vi "MT Compensate Sample Clock Frequency Error (QAM).vi"(0 "input complex waveform":T1={"t0"=0.0, "dt"=1.0, "Y"=[]} {"Y" format="%.3f"; "dt" format="%^.2e"; "t0" format="%.4f"}, 5 "samples per symbol":i32=16, 7 "matched filter coefficients":dbl[](array[numeric]), 9 "clock phase computation window (symbols)":i32=256, 11 "error in (no error)":errorcluster) -> (4 "output complex waveform":T1 {"Y" format="%.3f"; "dt" format="%^.2e"; "t0" format="%.4f"}, 6 "sample clock frequency error (ppm)":dbl, 15 "error out":errorcluster)   [LabVIEW 2020, in "niDMT.lvlib"]
doc: "This polymorphic instance corrects the sample clock frequency offset before calling the MT Demodulate QAM VI."
uses:
  <vilib>/addons/Modulation/niDMT.lvlib
  <vilib>/addons/Modulation/Analog/controls/Complex Data Waveform.ctl
  <vilib>/Analysis/baseanly.llb/Mean (DBL).vi
  <vilib>/addons/Modulation/Analog/support/Validators/mod_Fractional Resample Validate.vi
  <vilib>/addons/Modulation/Analog/support/Validators/mod_Check Flush State.vi
  <vilib>/addons/Modulation/Analog/support/mod_FractionalResampler.vi
  <vilib>/addons/Modulation/Analog/support/mod_Integer Rate Interpolation.vi
  <vilib>/addons/Modulation/Analog/support/mod_Set Error Source.vi
  <vilib>/addons/Modulation/Analog/support/Validators/mod_WFErrorHandler.vi
  <vilib>/addons/Modulation/Analog/support/mod_PerformResampling.vi
  <vilib>/Utility/error.llb/Error Cluster From Error Code.vi
  <vilib>/addons/Modulation/Analog/support/mod_Resampling Factors.vi
  <vilib>/addons/Modulation/Analog/support/mod_ResamplingFilter.vi
  <vilib>/addons/Modulation/Analog/support/mod_Generate Integer Interpolation Filter.vi
  <vilib>/addons/Modulation/Digital/General/MT Apply Matched Filter (Generic).vi
  <vilib>/addons/Modulation/niAMT.lvlib
  <vilib>/Analysis/NI_AALPro.lvlib
  <vilib>/Analysis/NI_AALBase.lvlib
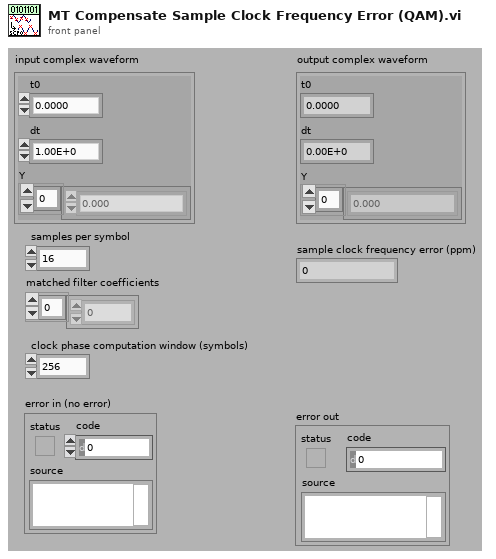
[diagram p1: front panel]
types:
  T1 = typedef "niAMT.lvlib/Complex Data Waveform.ctl" = cluster{"t0":dbl, "dt":dbl, "Y":cdb[]}
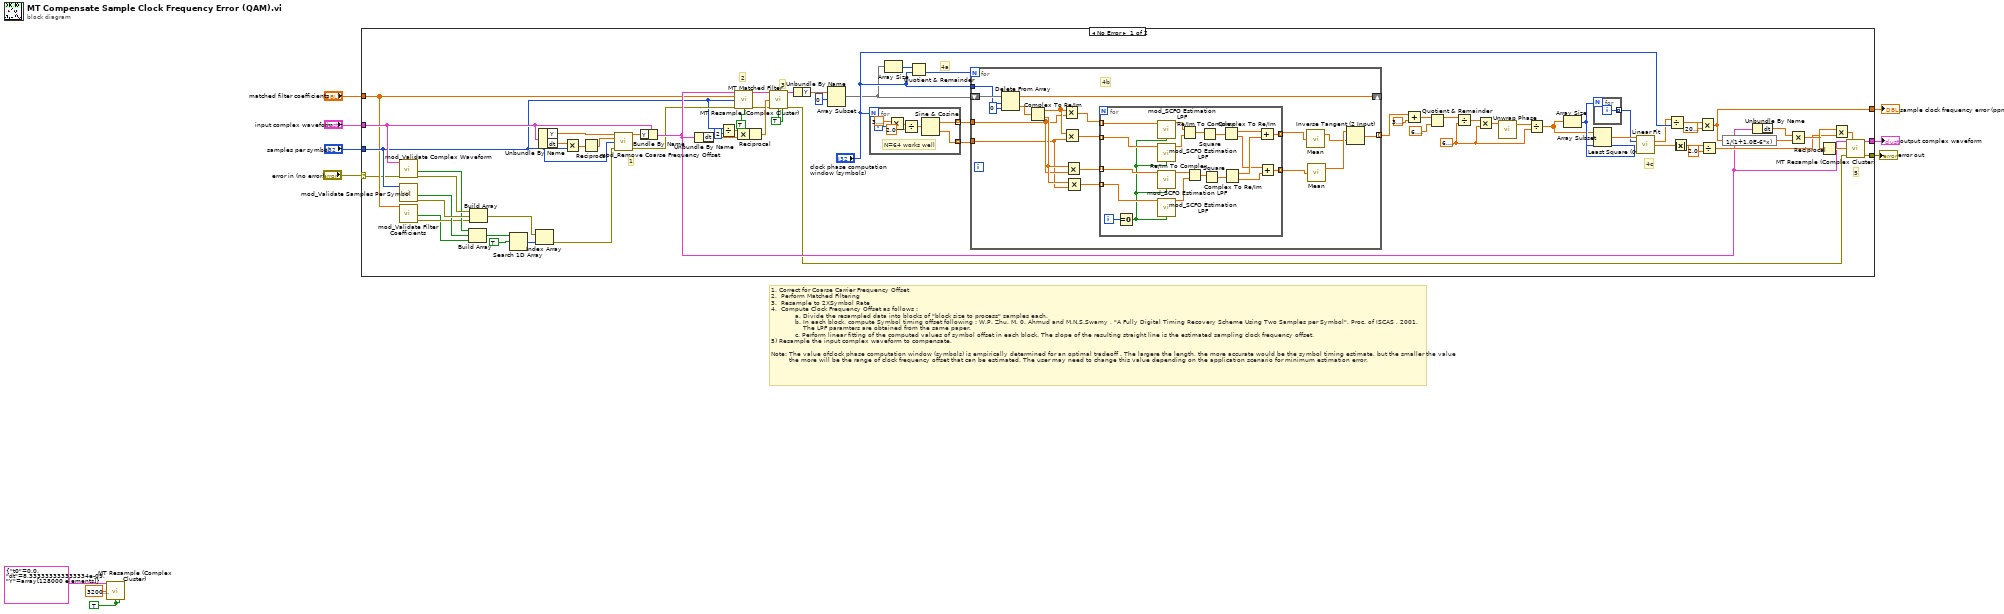
[diagram p0: block diagram]
diagram:
  w8 = TRUE ("reset? (T)")
  # "1.\tCorrect for Coarse Carrier Frequency Offset\n2.\t Perform Matched Filtering\n3. \tResample to 2XSymbol Rate\n4. \tCompute Clock Frequency Offset as follows : \n            a.\tDivide the resampled data into blocks of \"block size to process\" samples each. \n            b.\tIn each block, compute Symbol timing offset following : W.P. Zhu, M. 0. Ahmud and M.N.S.Swamy , \"A Fully Digital Timing Recovery Scheme Using Two Samples per Symbol\", Proc. of ISCAS , 2001. \n                The LPF paramters are obtained from the same paper. \n            c.\tPerform linear fitting of the computed values of symbol offset in each block. The slope of the resulting straight line is the estimated sampling clock frequency offset. \n5)\tResample the input complex waveform to compensate.\n\nNote: The value ofclock phase computation window (symbols) is empirically determined for an optimal tradeoff . The largere the length, the more accurate would be the symbol timing estimate, but the smaller the value \n         the more will be the range of clock frequency offset that can be estimated. The user may need to change this value depending on the application scenario for minimum estimation error."
  n1 = call <vilib>:"MT Resample (Complex Cluster).vi"("input complex waveform"=T1 {"t0"=0.0, "dt"=8.333333333333334e-09, "Y"=array[128000 elements]} ("IQ data (complex) in"), "desired sample rate (Hz)"=32000000.0, "reset? (T)"=w8, "flush buffers? (F)"=w8) -> ()  [unwired: 2 in, 10 out]
  n2 = case shown="No Error" "error in (no error)" {
    selector: "error in (no error)" -> [w12 w127]
    tunnel: [w44 _] -> w10
    tunnel: [w42 _] -> w7
    tunnel: "matched filter coefficients" -> [w13 _]
    tunnel: "input complex waveform" -> [w15 _]
    tunnel: "samples per symbol" -> [w14 _]
    tunnel: [w26 w127] -> w1
    frame No Error {
      w69 = u16 0 items=["Least Square", "Least Absolute Residual", "Bisquare"] ("method")
      w72 = 6.283185307179586
      w56 = TRUE ("reset? (T)")
      # "5"
      # "4c"
      # "4a"
      # "3"
      # "2"
      # "1"
      n3 = call <vilib>:"mod_Validate Complex Waveform.vi"("error in (no error)"=w12, "input complex waveform"=w15) -> ("error out"=w20:errorcluster, "error?"=w18:bool)  [unwired: 8 out]
      n4 = call <vilib>:"mod_Validate Samples Per Symbol.vi"("Samples Per Symbol"=w14) -> ("error out"=w21:errorcluster, "error?"=w19:bool)  [unwired: 9 out]
      n5 = call <vilib>:"mod_Validate Filter Coefficients.vi"("Filter Coefficients"=w13) -> ("error out"=w17:errorcluster, "error?"=w16:bool)  [unwired: 9 out]
      n6 = Build Array(w18, w19, w16) -> (w23:bool[])
      n7 = Build Array(w20, w21, w17) -> (w22:errorcluster[])
      n8 = Search 1D Array(1D array=w23, element=TRUE) -> (index of element=w25:i32)  [unwired: 1 out]
      n9 = Index Array(array=w22, index=w25) -> (element=w11:errorcluster)
      n10 = Unbundle By Name(w15) -> ("Y"=w35:cdb[], "dt"=w34:dbl)
      n11 = Multiply(x=w34, y=w14) -> (x*y=w33:dbl)
      n12 = Reciprocal(x=w33) -> (1/x=w32:dbl)
      n13 = call <vilib>:"mod_Remove Coarse Frequency Offset.vi"("Signal In"=w35, "Symbol Rate, Hz"=w32, "Samples Per Symbol (16)"=w14, "error in (no error)"=w11) -> ("Signal Out"=w31:cdb[], "error out"=w29:errorcluster)  [unwired: 4 in, 6 out]
      n14 = Bundle By Name(cluster=w15, "Y"=w31) -> (w30:T1)
      n15 = Unbundle By Name(w30) -> ("dt"=w53:dbl)
      n16 = Divide(x=w14, y=2) -> (x/y=w57:dbl)
      n17 = Multiply(x=w57, y=w53) -> (x*y=w52:dbl)
      n18 = call-poly <vilib>:"MT Matched Filter.vi"("input complex waveform"=w30, "matched filter coefficients"=w13, "samples per symbol (16)"=w14, "error in (no error)"=w29, "reset? (T)"=TRUE) -> ("output complex waveform"=w51:T1, "error out"=w28:errorcluster)  [unwired: 9 out]
      n19 = Reciprocal(x=w52) -> (1/x=w43:dbl)
      n20 = call <vilib>:"MT Resample (Complex Cluster).vi"("input complex waveform"=w51, "desired sample rate (Hz)"=w43, "error in (no error)"=w28, "reset? (T)"=w56, "flush buffers? (F)"=w56) -> ("output complex waveform"=w45:T1, "error out"=w27:errorcluster)  [unwired: 1 in, 8 out]
      n21 = Unbundle By Name(w45) -> ("Y"=w65:cdb[])
      n22 = Array Subset(array=w65, index=0) -> (w55:cdb[])  [unwired: 1 in]
      n23 = for {
        N: "clock phase computation window (symbols)" -> [_]
        tunnel: [w121] -> w78 mode=indexing
        tunnel: [w120] -> w59 mode=indexing
        i -> [w125]
        # "N=64 works well"
        n24 = Multiply(x=3.141592653589793, y=w125) -> (x*y=w124:dbl)
        n25 = Divide(x=w124, y=2.0) -> (x/y=w122:dbl)
        n26 = Sine & Cosine(0:w122) -> (1:w121:dbl, 2:w120:dbl)
      }
      n27 = Array Size(array=w55) -> (size(s)=w80:i32)
      n28 = Quotient & Remainder(x=w80, y="clock phase computation window (symbols)") -> (floor(x/y)=w79:i32)  [unwired: 1 out]
      n29 = for {
        N: w79 -> [_]
        shift-right: [w96] -> _
        shift-left: w55 -> [w99]
        tunnel: "clock phase computation window (symbols)" -> [w98]
        tunnel: w78 -> [w93]
        tunnel: w59 -> [w92]
        tunnel: [w83] -> w77 mode=indexing
        # "4b"
        n30 = Delete From Array(array=w99, length=w98, index=0) -> (deleted portion=w82:cdb[], array with subset deleted=w96:cdb[])
        n31 = Complex To Re/Im(x + iy=w82) -> (x=w95:dbl[], y=w94:dbl[])
        n32 = Multiply(x=w95, y=w93) -> (x*y=w91:dbl[])
        n33 = Multiply(x=w95, y=w92) -> (x*y=w90:dbl[])
        n34 = Multiply(x=w94, y=w93) -> (x*y=w89:dbl[])
        n35 = Multiply(x=w94, y=w92) -> (x*y=w88:dbl[])
        n36 = for {
          tunnel: w91 -> [w119] mode=indexing
          tunnel: w90 -> [w117] mode=indexing
          tunnel: w89 -> [w116] mode=indexing
          tunnel: w88 -> [w115] mode=indexing
          tunnel: [w101] -> w87 mode=indexing
          tunnel: [w100] -> w86 mode=indexing
          i -> [w118]
          n37 = Equal To 0?(x=w118) -> (x = 0?=w114:bool)
          n38 = call <vilib>:"mod_SCFO Estimation LPF.vi"("x[n]"=w119, "reset"=w114) -> ("y[n]"=w113:dbl)  [unwired: 13 out]
          n39 = call <vilib>:"mod_SCFO Estimation LPF.vi"("x[n]"=w117, "reset"=w114) -> ("y[n]"=w112:dbl)  [unwired: 13 out]
          n40 = call <vilib>:"mod_SCFO Estimation LPF.vi"("x[n]"=w116, "reset"=w114) -> ("y[n]"=w111:dbl)  [unwired: 13 out]
          n41 = call <vilib>:"mod_SCFO Estimation LPF.vi"("x[n]"=w115, "reset"=w114) -> ("y[n]"=w110:dbl)  [unwired: 13 out]
          n42 = Re/Im To Complex(1:w112, 2:w113) -> (0:w109:cdb)
          n43 = Re/Im To Complex(1:w110, 2:w111) -> (0:w108:cdb)
          n44 = Square(x=w109) -> (x^2=w107:cdb)
          n45 = Square(x=w108) -> (x^2=w106:cdb)
          n46 = Complex To Re/Im(x + iy=w107) -> (x=w105:dbl, y=w103:dbl)
          n47 = Complex To Re/Im(x + iy=w106) -> (x=w104:dbl, y=w102:dbl)
          n48 = Add(x=w105, y=w104) -> (x+y=w101:dbl)
          n49 = Add(x=w103, y=w102) -> (x+y=w100:dbl)
        }
        n50 = call-poly <vilib>:"Mean.vi"("X"=w87) -> ("mean"=w84:dbl)  [unwired: 1 out]
        n51 = call-poly <vilib>:"Mean.vi"("X"=w86) -> ("mean"=w85:dbl)  [unwired: 1 out]
        n52 = Inverse Tangent (2 Input)(1:w84, 2:w85) -> (0:w83:dbl)
      }
      n53 = Add(x=w77, y=3.141592653589793) -> (x+y=w62:dbl[])
      n54 = Quotient & Remainder(x=w62, y=6.283185307179586) -> (x-y*floor(x/y)=w61:dbl[])  [unwired: 1 out]
      n55 = Divide(x=w61, y=w72) -> (x/y=w60:dbl[])
      n56 = Multiply(x=w60, y=w72) -> (x*y=w74:dbl[])
      n57 = call <vilib>:"Unwrap Phase.vi"("Phase"=w74) -> ("Unwrapped Phase"=w73:dbl[])  [unwired: 1 in, 9 out]
      n58 = Divide(x=w73, y=w72) -> (x/y=w67:dbl[])
      n59 = Array Size(array=w67) -> (size(s)=w70:i32)
      n60 = for {
        N: w70 -> [_]
        tunnel: [w81] -> w68 mode=indexing
        i -> [w81]
      }
      n61 = Array Subset(array=w67, length=w70) -> (w71:dbl[])  [unwired: 1 in]
      n62 = call <vilib>:"Linear Fit.vi"("Y"=w71, "X"=w68, "method"=w69) -> ("slope"=w66:dbl, "intercept"=w40:dbl)  [unwired: 3 in, 8 out]
      n63 = Divide(x=w66, y="clock phase computation window (symbols)") -> (x/y=w50:dbl)
      n64 = Absolute Value(x=w40) -> (abs(x)=w39:dbl)
      n65 = Multiply(x=w50, y=2000000.0) -> (x*y=w44:dbl)
      n66 = Divide(x=w39, y=2.0) -> (x/y=w36:dbl)
      n67 = expression code="1/(1+1.0E-6*x)"(w44) -> (w47:dbl)
      n68 = Unbundle By Name(w30) -> ("dt"=w48:dbl)
      n69 = Multiply(x=w48, y=w47) -> (x*y=w37:dbl)
      n70 = Reciprocal(x=w37) -> (1/x=w46:dbl)
      n71 = Multiply(x=w37, y=w36) -> (x*y=w38:dbl)
      n72 = call <vilib>:"MT Resample (Complex Cluster).vi"("input complex waveform"=w30, "initial sample offset (sec)"=w38, "desired sample rate (Hz)"=w46, "error in (no error)"=w27) -> ("output complex waveform"=w42:T1, "error out"=w26:errorcluster)  [unwired: 2 in, 8 out]
    }
    frame Error {
    }
  }
  "sample clock frequency error (ppm)" <- w10
  "output complex waveform" <- w7
  "error out" <- w1
